vi "SInSubVI.vi"(6 "Error In":errorcluster, 8 "Frequency":dbl, 9 "DC Offset":dbl, 10 "Duty Cycle":dbl, 11 "Amplitude":dbl) -> (0 "Error Out":errorcluster, 3 "Array":dbl[](array[numeric]))   [LabVIEW 2017]
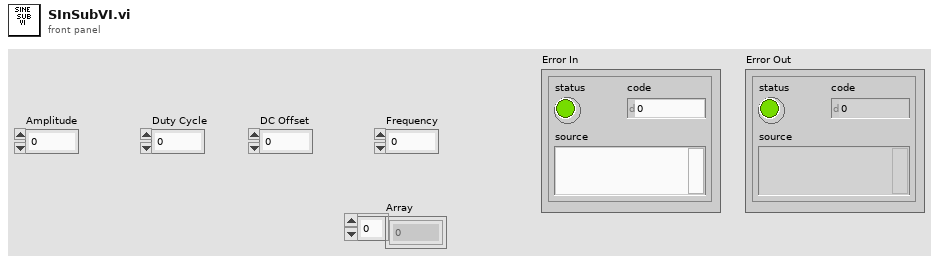
[diagram p1: front panel]
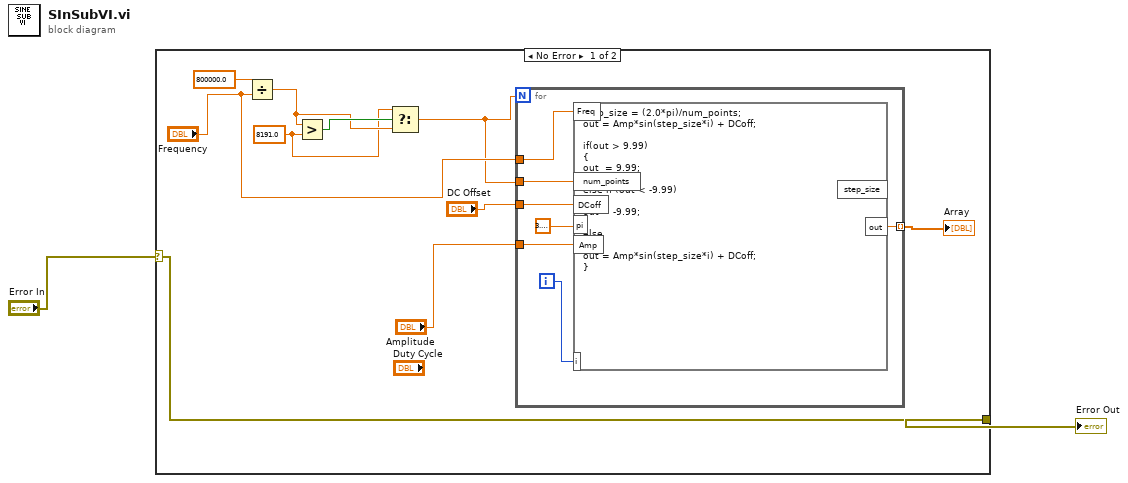
[diagram p0: block diagram]
diagram:
  n1 = case shown="No Error" "Error In" {
    selector: "Error In" -> [w12 w20]
    tunnel: [w12 w20] -> w1
    frame No Error {
      w5 = 8191.0 ("y")
      n2 = Divide(x=800000.0, y="Frequency") -> (x/y=w6:dbl)
      n3 = Greater?(x=w6, y=w5) -> (0:w8:bool)
      n4 = Select(t=w5, s=w8, f=w6) -> (s? t:f=w3:dbl)
      n5 = for {
        N: w3 -> [_]
        tunnel: [w18] -> w11 mode=indexing
        tunnel: "Amplitude" -> [w16]
        tunnel: "DC Offset" -> [w15]
        tunnel: "Frequency" -> [w14]
        tunnel: w3 -> [w13]
        i -> [w19]
        n6 = formula code="step_size = (2.0*pi)/num_points;\nout = Amp*sin(step_size*i) + DCoff;\n\nif(out > 9.99)\n{\nout  = 9.99;\n}\nelse if (out < -9.99)\n{\nout = -9.99;\n}\nelse\n{\nout = Amp*sin(step_size*i) + DCoff;\n}"("Freq"=w14, "DCoff"=w15, "Amp"=w16, "pi"=3.141592653589793, "i"=w19, "num_points"=w13) -> ("out"=w18:dbl)  [unwired: 1 out]
      }
      "Array" <- w11
    }
    frame Error {
    }
  }
  "Error Out" <- w1
